vi "SR830 Record to file.vi"() -> ()   [LabVIEW 2018]
doc: "This example shows how to configure the instrument to read all the parameters available."
uses:
  <instrlib>/Stanford Research 830/Public/Data/Read (All Parameters).vi
  <instrlib>/Stanford Research 830/Stanford Research 830.lvlib
panel:
  in  "Stop":bool
  out "Saving to:":string
  in  "Internal Reference Frequency (1000 Hz)":dbl=1000.0
  in  "Sine Output Amplitude (1 V)":dbl=1.0
  out "Parameter Values":T1
  in  "Sensitivity (26: 1 V/uA)":i16(ring)=26 items=["Auto Gain"=-1, "2 nV/fA"=0, "5 nV/fA"=1, "10 nV/fA"=2, "20 nV/fA"=3, "50 nV/fA"=4, "100 nV/fA"=5, "200 nV/fA"=6, "500 nV/fA"=7, "1 uV/pA"=8, "2 uV/pA"=9, "5 uV/pA"=10, "10 uV/pA"=11, "20 uV/pA"=12, "50 uV/pA"=13, "100 uV/pA"=14, "200 uV/pA"=15, "500 uV/pA"=16, "1 mV/nA"=17, "2 mV/nA"=18, "5 mV/nA"=19, "10 mV/nA"=20, "20 mV/nA"=21, "50 mV/nA"=22, "100 mV/nA"=23, "200 mV/nA"=24, "500 mV/mA"=25, "1 V/uA"=26]
  in  "Dynamic Reserve (2: Low Noise)":i16(ring)=2 items=["High Reserve"=0, "Normal"=1, "Low Noise"=2, "Auto Reserve"=-1]
  in  "Reference Source (1: Internal)":u16(ring)=1 items=["External", "Internal"]
  in  "Input Coupling (0: AC)":u16(ring) items=["AC", "DC"]
  in  "Input Connection (0: Single-Ended Voltage)":u16(ring) items=["Single-Ended Voltage", "Differential Voltage", "1 MOhm Current Gain", "100 MOhm Current Gain"]
  in  "VISA resource name":refnum<visa-resource-name>
  # "Save measurement from SR830 Lock-In"
  # "(c) 2006 National Instruments.  ALL RIGHTS RESERVED."
  # "SR830 Lock-In Amplifier Front Panel"
  # "This VI obtains a series of measurements from a Stanford SR830 lock-in amplifier\nand saves it to an LVM file chosen by the user."
  # "(GPIB0::9::INSTR)"
  # "Operating the VI"
  # "First set the amplifier parameters on the right, and then run the VI (press the arrow in the toolbar above or Ctrl-R).\n\nA prompt will appear asking you for a file name. If you choose an exisiting file, Labview will append data at the end of it.\n\nThe instrument then runs until you stop it on the button below:"
  # "Input Signal"
  # "Reference"
  # "Sensitivity and Reserve"
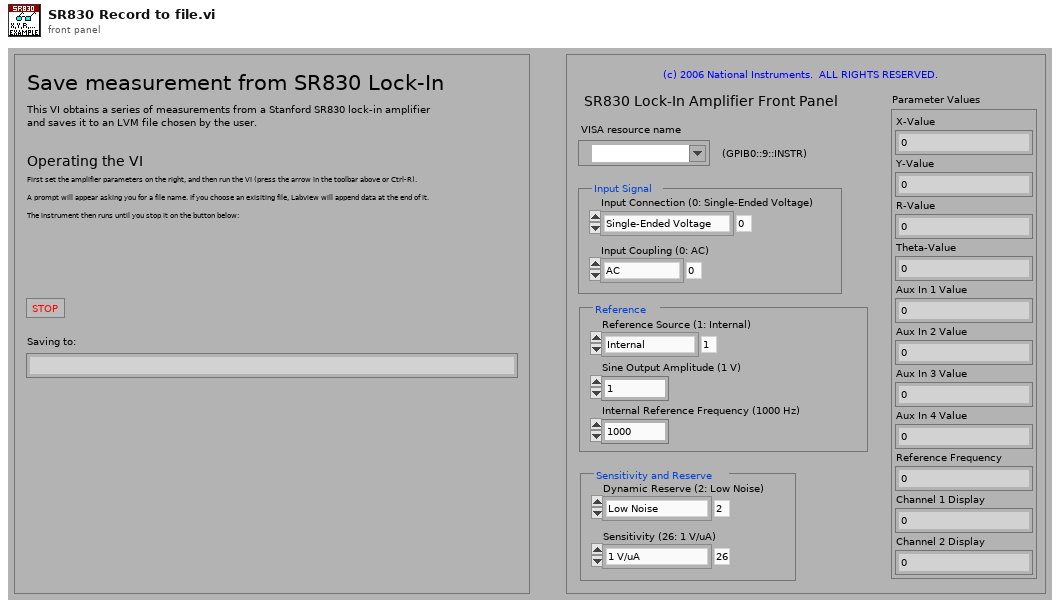
[diagram p1: front panel]
types:
  T1 = cluster{"X-Value":dbl, "Y-Value":dbl, "R-Value":dbl, "Theta-Value":dbl, "Aux In 1 Value":dbl, "Aux In 2 Value":dbl, "Aux In 3 Value":dbl, "Aux In 4 Value":dbl, "Reference Frequency":dbl, "Channel 1 Display":dbl, "Channel 2 Display":dbl}
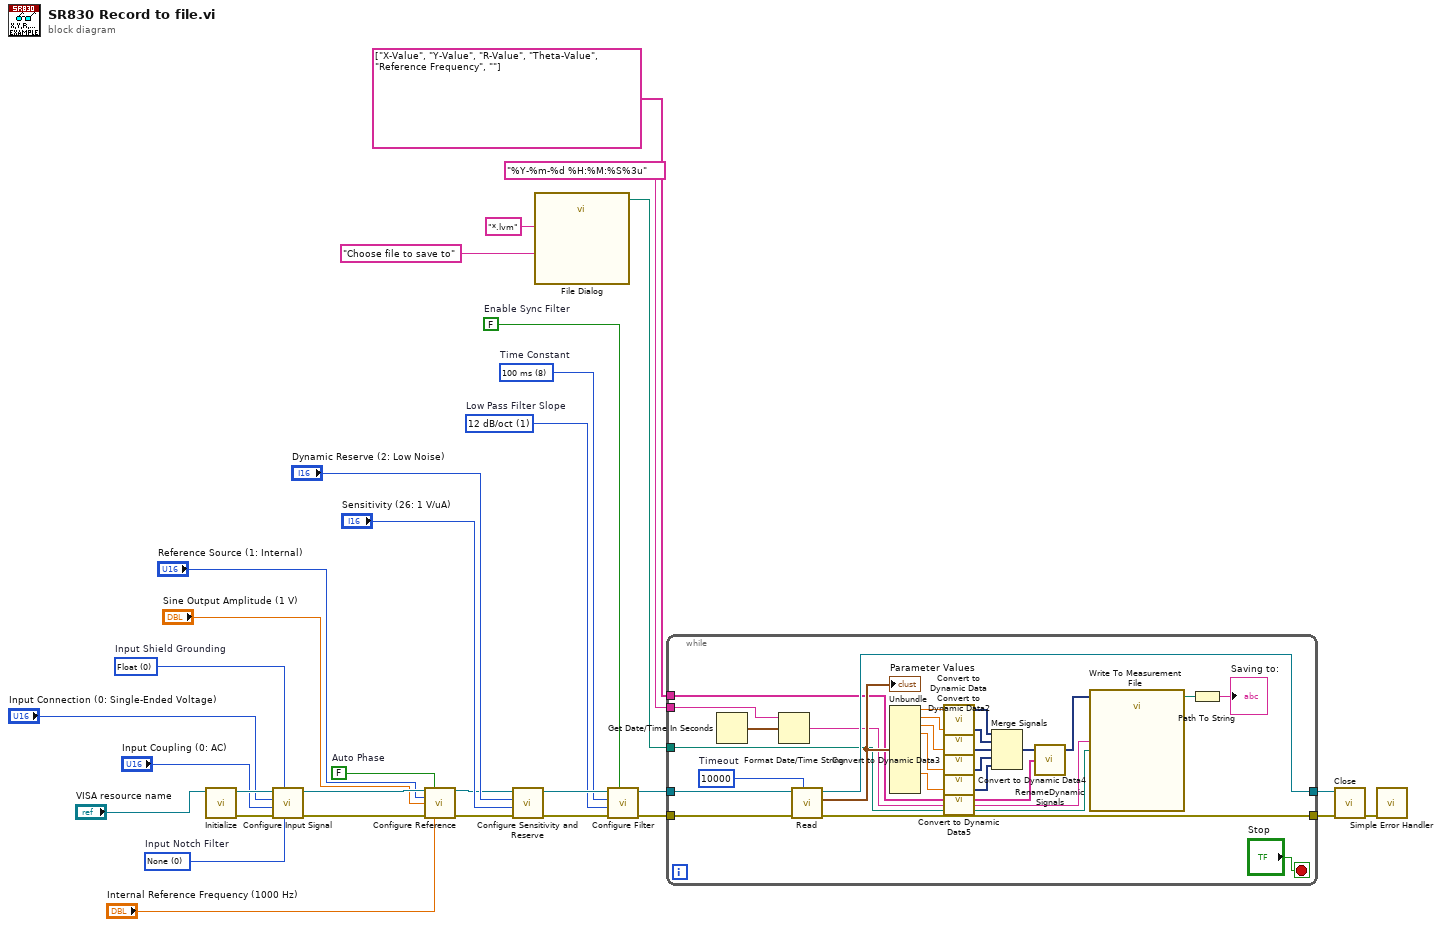
[diagram p0: block diagram]
diagram:
  w10 = FALSE  # Enable Sync Filter
  w11 = u16 1 items=["6 dB/oct", "12 dB/oct", "18 db/oct", "24 dB/oct"]  # Low Pass Filter Slope
  w12 = u16 8 items=["10 us", "30 us", "100 us", "300 us", "1 ms", "3 ms", "10 ms", "30 ms", "100 ms", "300 ms", "1 s", "3 s", "10 s", "30 s", "100 s", "300 s", "1 ks", "3 ks", "10 ks", "30 ks"]  # Time Constant
  w22 = FALSE  # Auto Phase
  w23 = u16 0 items=["None", "Line Notch", "2x Line Notch", "Both Notch Filters"]  # Input Notch Filter
  w24 = u16 0 items=["Float", "Ground"]  # Input Shield Grounding
  n1 = call <instrlib>:"Initialize.vi"("VISA resource name"="VISA resource name") -> ("error out"=w31:errorcluster, "VISA resource name out"=w30:refnum<visa-resource-name>)  [unwired: 9 in]
  n2 = call <instrlib>:"Configure Input Signal.vi"("Input Notch Filter (0: None)"=w23, "Input Shield Grounding (0: Float)"=w24, "error in (no error)"=w31, "Input Coupling (0: AC)"="Input Coupling (0: AC)", "Input Connection (0: Single-Ended Voltage)"="Input Connection (0: Single-Ended Voltage)", "VISA resource name"=w30) -> ("error out"=w28:errorcluster, "VISA resource name out"=w29:refnum<visa-resource-name>)  [unwired: 4 in]
  n3 = call <instrlib>:"Configure Reference.vi"("VISA resource name"=w29, "Auto Phase (T: Enabled)"=w22, "Reference Source (1: Internal)"="Reference Source (1: Internal)", "Sine Output Amplitude (1 V)"="Sine Output Amplitude (1 V)", "error in (no error)"=w28, "Internal Reference Frequency (1000 Hz)"="Internal Reference Frequency (1000 Hz)") -> ("VISA resource name out"=w19:refnum<visa-resource-name>, "error out"=w18:errorcluster)  [unwired: 8 in]
  n4 = call <instrlib>:"Configure Sensitivity and Reserve.vi"("error in (no error)"=w18, "Sensitivity (-1: Auto gain)"="Sensitivity (26: 1 V/uA)", "Dynamic Reserve (-1: Auto Reserve)"="Dynamic Reserve (2: Low Noise)", "VISA resource name"=w19) -> ("error out"=w13:errorcluster, "VISA resource name out"=w14:refnum<visa-resource-name>)  [unwired: 6 in]
  n5 = call "File Dialog"("prompt"="Choose file to save to", "pattern (all files)"="*.lvm") -> ("selected path"=w3:path)  [unwired: 10 in, 3 out]
  n6 = call <instrlib>:"Configure Filter.vi"("Enable Sync Filter (F: Disable)"=w10, "error in (no error)"=w13, "Low Pass Filter Slope (1: 12dB/oct)"=w11, "Time Constant (8: 100ms)"=w12, "VISA resource name"=w14) -> ("error out"=w7:errorcluster, "VISA resource name out"=w6:refnum<visa-resource-name>)  [unwired: 5 in]
  n7 = while {
    tunnel: w7 -> [w58]
    tunnel: w6 -> [w57]
    tunnel: [w56] -> w5
    tunnel: [w55] -> w4
    tunnel: w3 -> [w51]
    tunnel: string[] ["X-Value", "Y-Value", "R-Value", "Theta-Value", "Reference Frequency", ""] -> [w50]
    tunnel: "%Y-%m-%d %H:%M:%S%3u" -> [w35]
    stop <- "Stop" stop-if-true
    w54 = u32 10000  # Timeout
    n8 = Get Date/Time In Seconds() -> (seconds since 1Jan1904=w34:timestamp)
    n9 = Format Date/Time String(time format string (%c)=w35, seconds (now)=w34) -> (date/time string=w33:string)  [unwired: 1 in]
    n10 = call-poly <instrlib>:"Read.vi"("Timeout (10000 ms)"=w54, "error in (no error)"=w58, "VISA resource name"=w57) -> ("error out"=w56:errorcluster, "Parameter Values"=w53:T1, "VISA resource name out"=w55:refnum<visa-resource-name>)  [unwired: 6 in]
    "Parameter Values" <- w53
    n11 = Unbundle(w53) -> ("X-Value"=w46:dbl, "Y-Value"=w45:dbl, "R-Value"=w44:dbl, "Theta-Value"=w43:dbl, "Reference Frequency"=w42:dbl)  [unwired: 6 out]
    n12 = call "Convert to Dynamic Data"("Double"=w46) -> ("Dynamic Data Type"=w36:dynamicdata)  [unwired: 3 in]
    n13 = call "Convert to Dynamic Data2"("Double"=w45) -> ("Dynamic Data Type"=w37:dynamicdata)  [unwired: 3 in]
    n14 = call "Convert to Dynamic Data3"("Double"=w44) -> ("Dynamic Data Type"=w38:dynamicdata)  [unwired: 3 in]
    n15 = call "Convert to Dynamic Data4"("Double"=w43) -> ("Dynamic Data Type"=w39:dynamicdata)  [unwired: 3 in]
    n16 = call "Convert to Dynamic Data5"("Double"=w42) -> ("Dynamic Data Type"=w40:dynamicdata)  [unwired: 3 in]
    n17 = Merge Signals(w36, w37, w38, w39, w40) -> (w41:dynamicdata)
    n18 = call "RenameDynamicSignals.vi"("New Signal Names"=w50, "Dynamic Data In"=w41) -> ("Dynamic Data Out"=w49:dynamicdata)  [unwired: 2 in, 1 out]
    n19 = call "Write To Measurement File"("Signals"=w49, "Filename"=w51, "Comment"=w33) -> ("Filename Out"=w47:path)  [unwired: 14 in, 2 out]
    n20 = Path To String(path=w47) -> (string=→"Saving to:":string)
  }
  n21 = call <instrlib>:"Close.vi"("error in (no error)"=w5, "VISA resource name"=w4) -> ("error out"=w27:errorcluster)  [unwired: 9 in]
  n22 = call <vilib>:"Simple Error Handler.vi"("error in (no error)"=w27) -> ()  [unwired: 4 in, 5 out]
